vi "PLC_logic_New.vi"(7 "Trigger":bool[](array[boolean]), 8 "IsActive?":bool, 9 "Inputs past":bool[](array[boolean]), 10 "Inputs":bool[](array[boolean]), 11 "Outputs past":bool[](array[boolean])) -> (0 "Output Data":u16, 1 "Inputs to save":bool[](array[boolean]), 2 "Outputs OUT":bool[](array[boolean]), 6 "Outputs to card":string[](array[string]))   [LabVIEW 2017]
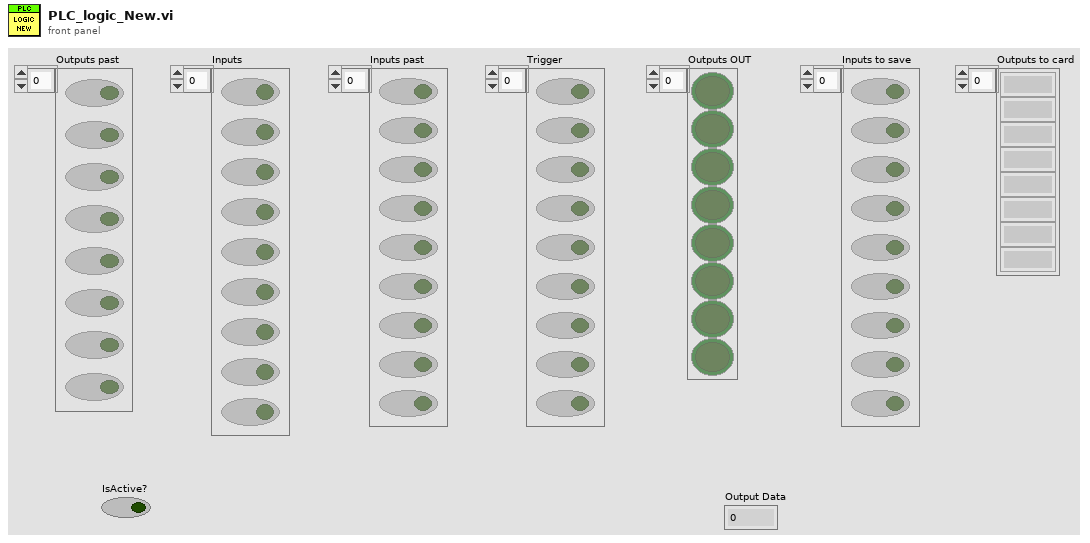
[diagram p1: front panel]
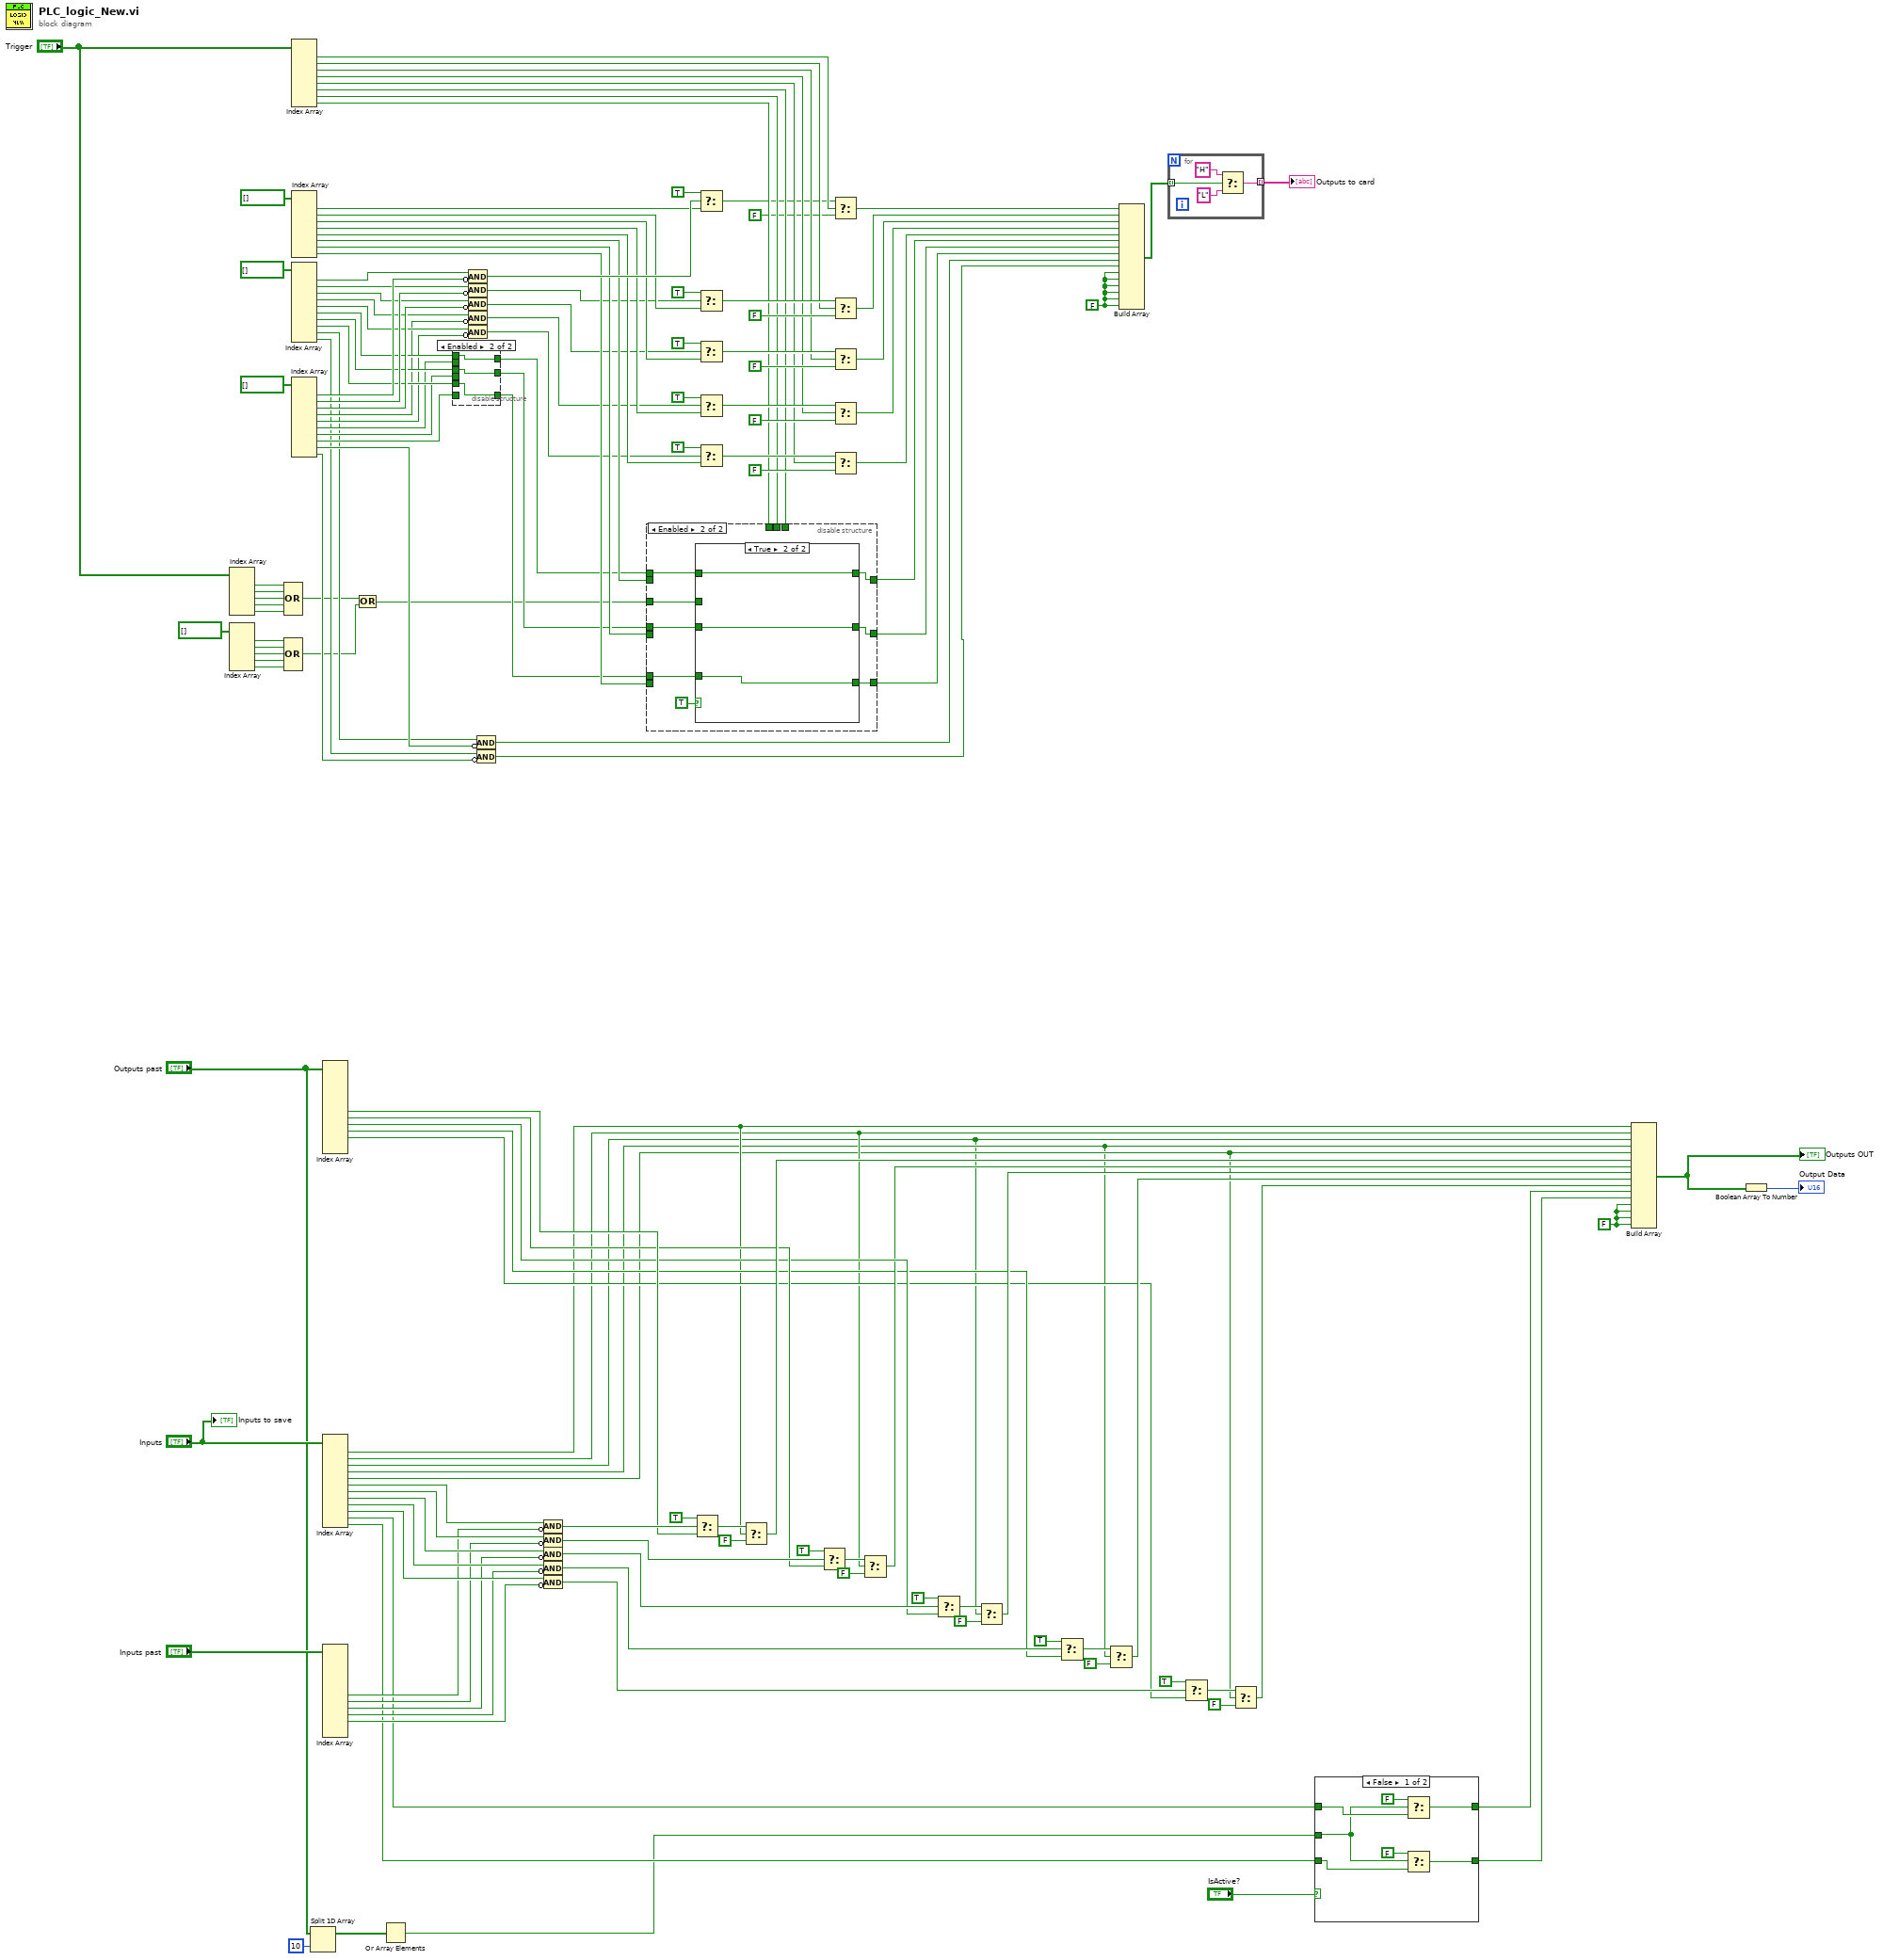
[diagram p0: block diagram]
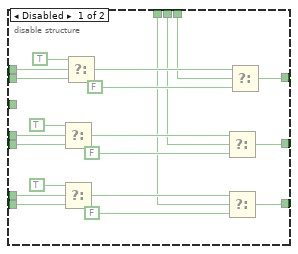
[diagram p3: hidden frame]
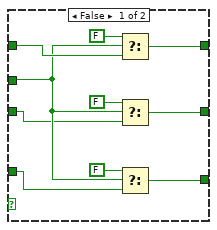
[diagram p4: hidden frame]
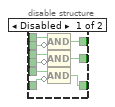
[diagram p5: hidden frame]
diagram:
  w17 = FALSE ("element")
  w65 = FALSE ("element")
  n1 = Index Array(array="Trigger") -> (element #1=w75:bool, element #2=w79:bool, element #3=w78:bool, element #4=w77:bool, element #5=w76:bool)  [unwired: 5 in]
  n2 = Index Array(array=bool[] []) -> (element #1=w69:bool, element #2=w80:bool, element #3=w81:bool, element #4=w82:bool, element #5=w83:bool)  [unwired: 5 in]
  n3 = Compound Arithmetic op=OR(w75, w79, w78, w77, w76) -> (w73:bool)
  n4 = Compound Arithmetic op=OR(w69, w80, w81, w82, w83) -> (w72:bool)
  n5 = Index Array(array=bool[] []) -> (element #1=w71:bool, element #2=w147:bool, element #3=w145:bool, element #4=w143:bool, element #5=w142:bool, element #6=w141:bool, element #7=w140:bool, element #8=w139:bool, element #9=w86:bool, element #10=w87:bool)  [unwired: 10 in]
  n6 = Index Array(array=bool[] []) -> (element #1=w148:bool, element #2=w146:bool, element #3=w144:bool, element #4=w138:bool, element #5=w137:bool, element #6=w136:bool, element #7=w135:bool, element #8=w134:bool, element #9=w88:bool, element #10=w89:bool)  [unwired: 10 in]
  n7 = Index Array(array="Trigger") -> (element #1=w132:bool, element #2=w96:bool, element #3=w95:bool, element #4=w94:bool, element #5=w93:bool, element #6=w92:bool, element #7=w91:bool, element #8=w90:bool)  [unwired: 8 in]
  n8 = Index Array(array=bool[] []) -> (element #1=w130:bool, element #2=w110:bool, element #3=w109:bool, element #4=w108:bool, element #5=w107:bool, element #6=w106:bool, element #7=w105:bool, element #8=w104:bool)  [unwired: 8 in]
  n9 = Split 1D Array(array="Outputs past", index=10) -> (first subarray=w2:bool[])  [unwired: 1 out]
  n10 = Index Array(array="Outputs past") -> (element #6=w44:bool, element #7=w25:bool, element #8=w24:bool, element #9=w19:bool, element #10=w18:bool)  [unwired: 12 in, 7 out]
  n11 = Index Array(array="Inputs") -> (element #1=w14:bool, element #2=w13:bool, element #3=w10:bool, element #4=w11:bool, element #5=w12:bool, element #6=w57:bool, element #7=w56:bool, element #8=w55:bool, element #9=w54:bool, element #10=w53:bool, element #11=w7:bool, element #12=w6:bool)  [unwired: 12 in]
  n12 = Index Array(array="Inputs past") -> (element #6=w52:bool, element #7=w51:bool, element #8=w50:bool, element #9=w49:bool, element #10=w48:bool)  [unwired: 12 in, 7 out]
  n13 = Or(x=w73, y=w72) -> (x .or. y?=w70:bool)
  n14 = Or Array Elements(Boolean array=w2) -> (logical OR=w1:bool)
  n15 = disable-structure shown="Enabled" {
    disable-tunnel: w141 -> [w158 w161]
    disable-tunnel: w140 -> [w157 w160]
    disable-tunnel: w139 -> [w156 w159]
    disable-tunnel: w136 -> [w155 _]
    disable-tunnel: w135 -> [w154 _]
    disable-tunnel: w134 -> [w153 _]
    disable-tunnel: [w152 w159] -> w103
    disable-tunnel: [w151 w160] -> w102
    disable-tunnel: [w150 w161] -> w101
    frame Disabled {
      n16 = Compound Arithmetic op=AND(w158, invert w155) -> (w150:bool)
      n17 = Compound Arithmetic op=AND(w157, invert w154) -> (w151:bool)
      n18 = Compound Arithmetic op=AND(w156, invert w153) -> (w152:bool)
    }
    frame Enabled {
    }
  }
  n19 = Compound Arithmetic op=AND(w71, invert w148) -> (w133:bool)
  n20 = Compound Arithmetic op=AND(w147, invert w146) -> (w97:bool)
  n21 = Compound Arithmetic op=AND(w145, invert w144) -> (w98:bool)
  n22 = Compound Arithmetic op=AND(w143, invert w138) -> (w99:bool)
  n23 = Compound Arithmetic op=AND(w142, invert w137) -> (w100:bool)
  n24 = Compound Arithmetic op=AND(w86, invert w88) -> (w85:bool)
  n25 = Compound Arithmetic op=AND(w87, invert w89) -> (w84:bool)
  n26 = Compound Arithmetic op=AND(w57, invert w52) -> (w45:bool)
  n27 = Compound Arithmetic op=AND(w56, invert w51) -> (w29:bool)
  n28 = Compound Arithmetic op=AND(w55, invert w50) -> (w28:bool)
  n29 = Compound Arithmetic op=AND(w54, invert w49) -> (w27:bool)
  n30 = Compound Arithmetic op=AND(w53, invert w48) -> (w26:bool)
  n31 = disable-structure shown="Enabled" {
    disable-tunnel: [w173 w190] -> w113
    disable-tunnel: [w172 w188] -> w112
    disable-tunnel: [w171 w186] -> w111
    disable-tunnel: w106 -> [w170 _]
    disable-tunnel: w105 -> [w169 _]
    disable-tunnel: w104 -> [w168 _]
    disable-tunnel: w103 -> [w167 w185]
    disable-tunnel: w102 -> [w166 w187]
    disable-tunnel: w101 -> [w165 w189]
    disable-tunnel: w92 -> [w164 _]
    disable-tunnel: w91 -> [w163 _]
    disable-tunnel: w90 -> [w162 _]
    disable-tunnel: w70 -> [_ w184]
    frame Disabled {
      n32 = Select(t=TRUE ("f"), s=w166, f=w169) -> (s? t:f=w181:bool)
      n33 = Select(t=TRUE ("f"), s=w167, f=w168) -> (s? t:f=w175:bool)
      n34 = Select(t=TRUE ("f"), s=w165, f=w170) -> (s? t:f=w178:bool)
      n35 = Select(t=w181, s=w163, f=FALSE) -> (s? t:f=w172:bool)
      n36 = Select(t=w175, s=w162, f=FALSE) -> (s? t:f=w171:bool)
      n37 = Select(t=w178, s=w164, f=FALSE) -> (s? t:f=w173:bool)
    }
    frame Enabled {
      n38 = case shown="True" TRUE {
        tunnel: [w198 w203] -> w190
        tunnel: w189 -> [w200 w203]
        tunnel: [w195 w202] -> w188
        tunnel: w187 -> [w193 w202]
        tunnel: [w191 w201] -> w186
        tunnel: w185 -> [w192 w201]
        tunnel: w184 -> [w194 _]
        frame False {
          n39 = Select(t=FALSE, s=w194, f=w200) -> (s? t:f=w198:bool)
          n40 = Select(t=FALSE, s=w194, f=w193) -> (s? t:f=w195:bool)
          n41 = Select(t=FALSE, s=w194, f=w192) -> (s? t:f=w191:bool)
        }
        frame True {
        }
      }
    }
  }
  n42 = Select(t=TRUE, s=w45, f=w44) -> (s? t:f=w43:bool)
  n43 = Select(t=TRUE ("f"), s=w133, f=w130) -> (s? t:f=w67:bool)
  n44 = Select(t=TRUE ("f"), s=w97, f=w110) -> (s? t:f=w128:bool)
  n45 = Select(t=TRUE ("f"), s=w98, f=w109) -> (s? t:f=w125:bool)
  n46 = Select(t=TRUE ("f"), s=w99, f=w108) -> (s? t:f=w122:bool)
  n47 = Select(t=TRUE ("f"), s=w100, f=w107) -> (s? t:f=w119:bool)
  n48 = Select(t=w43, s=w14, f=FALSE) -> (s? t:f=w42:bool)
  n49 = Select(t=TRUE, s=w29, f=w25) -> (s? t:f=w41:bool)
  n50 = Select(t=w67, s=w132, f=FALSE) -> (s? t:f=w131:bool)
  n51 = Select(t=w128, s=w96, f=FALSE) -> (s? t:f=w117:bool)
  n52 = Select(t=w125, s=w95, f=FALSE) -> (s? t:f=w116:bool)
  n53 = Select(t=w122, s=w94, f=FALSE) -> (s? t:f=w115:bool)
  n54 = Select(t=w119, s=w93, f=FALSE) -> (s? t:f=w114:bool)
  n55 = Select(t=w41, s=w13, f=FALSE) -> (s? t:f=w23:bool)
  n56 = Select(t=TRUE, s=w28, f=w24) -> (s? t:f=w36:bool)
  n57 = Select(t=w36, s=w10, f=FALSE) -> (s? t:f=w22:bool)
  n58 = Select(t=TRUE, s=w27, f=w19) -> (s? t:f=w35:bool)
  n59 = Select(t=w35, s=w11, f=FALSE) -> (s? t:f=w21:bool)
  n60 = Build Array(w131, w117, w116, w115, w114, w113, w112, w111, w85, w84, w65, w65, w65, w65, w65, w65) -> (w16:bool[])
  n61 = for {
    tunnel: w16 -> [w205] mode=indexing
    tunnel: [w204] -> w149 mode=indexing
    n62 = Select(t="H", s=w205, f="L") -> (s? t:f=w204:string)
  }
  "Outputs to card" <- w149
  n63 = Select(t=TRUE, s=w26, f=w18) -> (s? t:f=w30:bool)
  n64 = Select(t=w30, s=w12, f=FALSE) -> (s? t:f=w20:bool)
  n65 = case shown="False" "IsActive?" {
    tunnel: [w212 w216] -> w9
    tunnel: w7 -> [w214 w216]
    tunnel: [w210 w215] -> w8
    tunnel: w6 -> [w208 w215]
    tunnel: w1 -> [w209 _]
    frame False {
      n66 = Select(t=FALSE, s=w209, f=w214) -> (s? t:f=w212:bool)
      n67 = Select(t=FALSE, s=w209, f=w208) -> (s? t:f=w210:bool)
    }
    frame True {
    }
  }
  n68 = Build Array(w14, w13, w10, w11, w12, w42, w23, w22, w21, w20, w9, w8, w17, w17, w17, w17) -> (w15:bool[])
  "Outputs OUT" <- w15
  n69 = Boolean Array To Number(Boolean array=w15) -> (number=→"Output Data":u16)
  "Inputs to save" <- "Inputs"
